vi "BASE.Device.ReadDeviceState.vi"(8 "error in (no error)":errorcluster, 10 "Timeout (5000 ms)":i32, 11 "Device.Simulation in":refnum<class "Device.Simulation.lvclass">) -> (0 "error out":errorcluster, 2 "Device State":variant, 3 "Device.Simulation out":refnum<class "Device.Simulation.lvclass">)   [LabVIEW 2019, in "Device.Simulation.lvlib" / "Device.Simulation.lvclass"]
uses:
  Device.Simulation.lvclass
  state--cluster.ctl
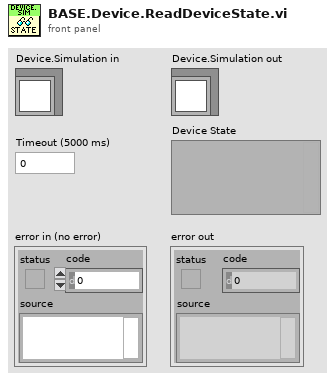
[diagram p1: front panel]
types:
  T1 = typedef "Device.Simulation.lvlib/Device.Simulation.lvclass/state--cluster.ctl" = cluster{"A1":dbl, "A2":dbl, "A3":dbl, "D1":bool, "D2":bool, "D3":bool}
  T2 = typedef "Device.Simulation.lvlib/Device.Simulation.lvclass/config--cluster.ctl" = cluster{"Name":string, "Time to Connect (ms)":u32, "Time to Check Connection (ms)":u32, "Time to Disconnect (ms)":u32, "Time to Read State (ms)":u32}
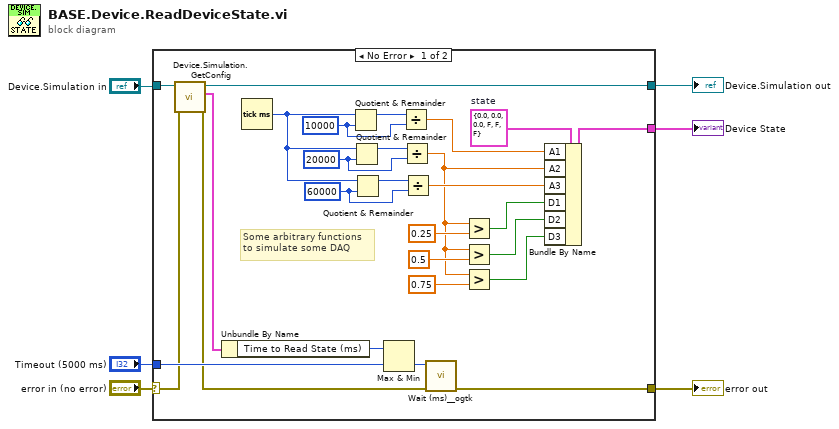
[diagram p0: block diagram]
diagram:
  n1 = case shown="No Error" "error in (no error)" {
    selector: "error in (no error)" -> [w10 w35]
    tunnel: [w33 w35] -> w2
    tunnel: "Device.Simulation in" -> [w12 w34]
    tunnel: [w11 w34] -> w3
    tunnel: "Timeout (5000 ms)" -> [w30 _]
    tunnel: [w13 _] -> w1
    frame No Error {
      w7 = T1 {"A1"=0.0, "A2"=0.0, "A3"=0.0, "D1"=FALSE, "D2"=FALSE, "D3"=FALSE}  # state
      w24 = u32 60000 ("y")
      w27 = u32 20000 ("y")
      w28 = u32 10000 ("y")
      # "Some arbitrary functions\nto simulate some DAQ"
      n2 = call "Device.Simulation.GetConfig.vi"("error in (no error)"=w10, "Device.Simulation in"=w12) -> ("error out"=w9:errorcluster, "config"=w8:T2, "Device.Simulation out"=w11:refnum<class "Device.Simulation.lvclass">)  [unwired: 7 in]
      n3 = Unbundle By Name(w8) -> ("Time to Read State (ms)"=w31:u32)
      n4 = Tick Count (ms)() -> (millisecond timer value=w23:u32)
      n5 = Quotient & Remainder(x=w23, y=w28) -> (x-y*floor(x/y)=w29:u32)  [unwired: 1 out]
      n6 = Quotient & Remainder(x=w23, y=w27) -> (x-y*floor(x/y)=w26:u32)  [unwired: 1 out]
      n7 = Quotient & Remainder(x=w23, y=w24) -> (x-y*floor(x/y)=w25:u32)  [unwired: 1 out]
      n8 = Max & Min(x=w31, y=w30) -> (min(x,y)=w32:u32)  [unwired: 1 out]
      n9 = Divide(x=w29, y=w28) -> (x/y=w21:dbl)
      n10 = Divide(x=w26, y=w27) -> (x/y=w16:dbl)
      n11 = Divide(x=w25, y=w24) -> (x/y=w22:dbl)
      n12 = call <userlib>:"Wait (ms)__ogtk.vi"("error in (no error)"=w9, "milliseconds to wait"=w32) -> ("error out"=w33:errorcluster)  [unwired: 8 in, 1 out]
      n13 = Greater?(x=w16, y=0.25) -> (0:w19:bool)
      n14 = Greater?(x=w16, y=0.5) -> (0:w15:bool)
      n15 = Greater?(x=w16, y=0.75) -> (0:w14:bool)
      n16 = Bundle By Name(cluster=w7, "A1"=w21, "A2"=w16, "A3"=w22, "D1"=w19, "D2"=w15, "D3"=w14) -> (w13:T1)
    }
    frame Error {
    }
  }
  "error out" <- w2
  "Device.Simulation out" <- w3
  "Device State" <- w1
